vi "Dialogue - Correct TimeStamp.vi"(8 "error in (no error)":errorcluster, 10 "Footer Text":string) -> (0 "error out":errorcluster)   [LabVIEW 2018, in "Receipt Parsing.lvlib"]
uses:
  Receipt Parsing.lvlib
panel:
  out "Footer Text":string
  # "DateTime did not parse. Please input manually using Footer Text as your guide."
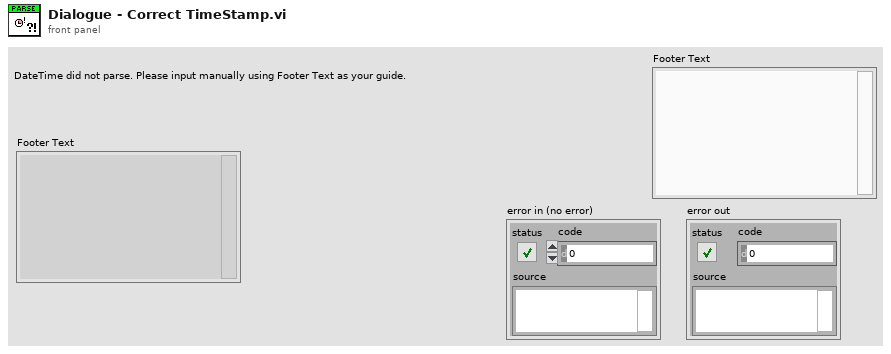
[diagram p1: front panel]
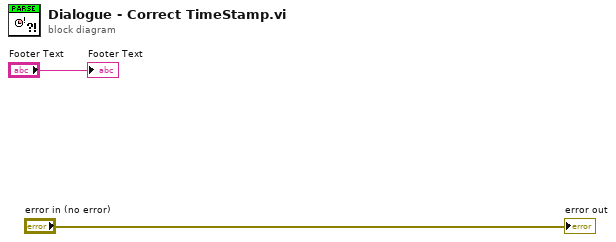
[diagram p0: block diagram]
diagram:
  "error out" <- "error in (no error)"
  "Footer Text" <- "Footer Text"
